vi "Read out VSET.vi"(4 "get more?":bool, 5 "All Channels (T)":bool=TRUE, 7 "Channel":u8, 8 "error in (no error)":errorcluster, 11 "BoardHandle":T2) -> (0 "error out":errorcluster, 1 "VSet constants":T1(array[cluster]), 2 "Vset values (V)":dbl[](array[numeric]) format="%.1f", 3 "BoardHandle out":T2)   [LabVIEW 2020, in "CAEN PSM.lvlib"]
doc: "This function returns VSet value"
uses:
  CAEN PSM.lvlib
  Private/BoardHandle.ctl
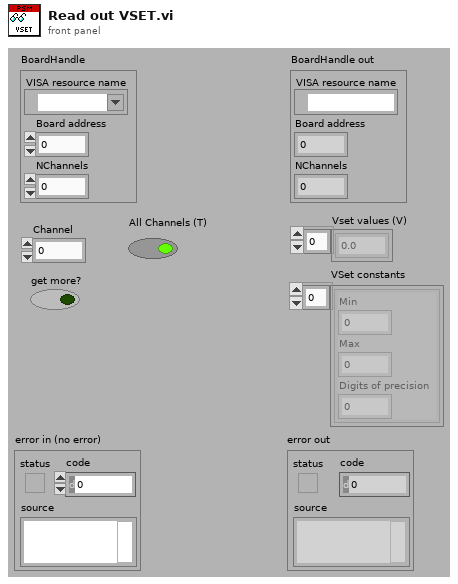
[diagram p1: front panel]
types:
  T1 = cluster{"Min":dbl, "Max":dbl, "Digits of precision":i32}[]
  T2 = typedef "CAEN PSM.lvlib/BoardHandle.ctl" = cluster{"VISA resource name":refnum<visa-resource-name>, "Board address":i8, "NChannels":u8}
  T3 = cluster{"Min":dbl, "Max":dbl, "Digits of precision":i32}
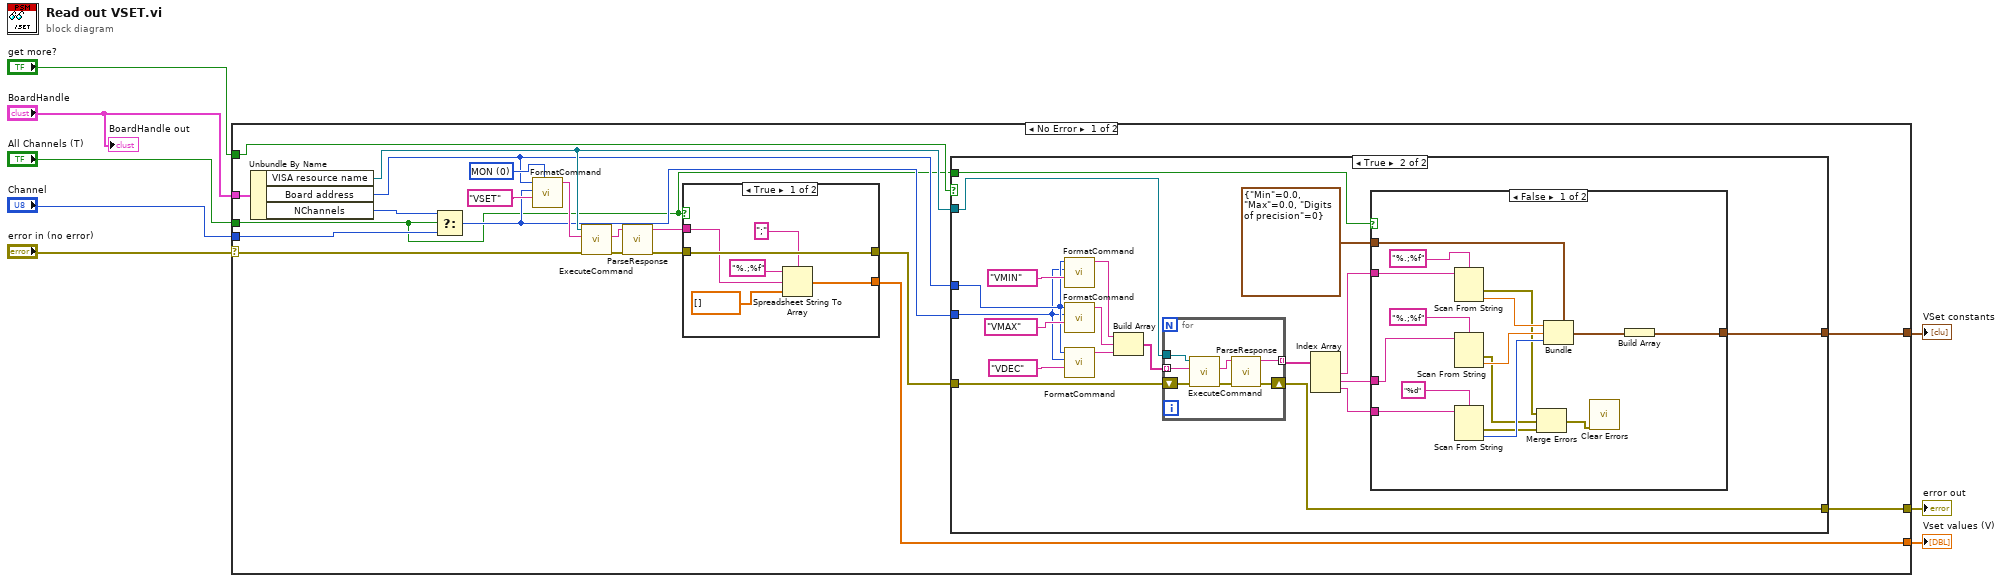
[diagram p0: block diagram]
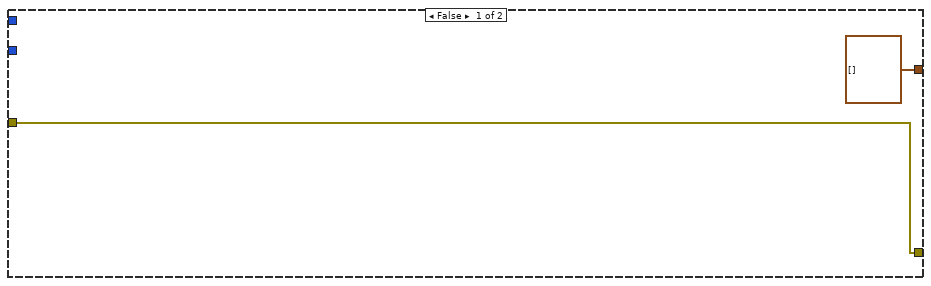
[diagram p2: hidden frame]
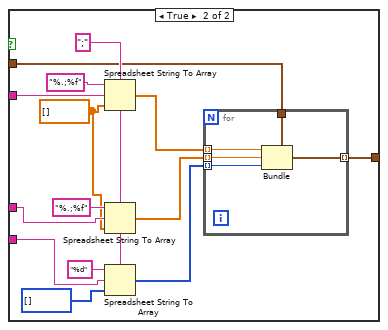
[diagram p3: hidden frame]
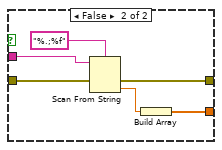
[diagram p4: hidden frame]
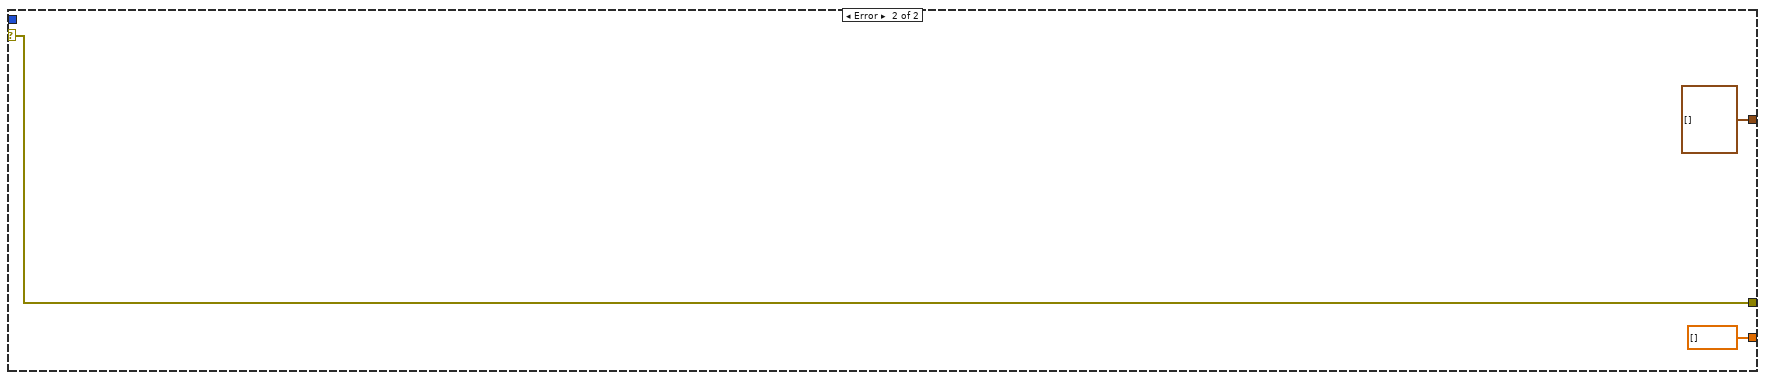
[diagram p5: hidden frame]
diagram:
  n1 = case shown="No Error" "error in (no error)" {
    selector: "error in (no error)" -> [w22 w106]
    tunnel: "All Channels (T)" -> [w9 _]
    tunnel: "Channel" -> [w27 _]
    tunnel: [w14 w106] -> w5
    tunnel: "BoardHandle" -> [w23 _]
    tunnel: [w17 dbl[] [] ("Trip value(s) s")] -> w3
    tunnel: "get more?" -> [w16 _]
    tunnel: [w10 T1 []] -> w1
    frame No Error {
      w28 = u8 0 items=["MON", "SET"] ("CMD")
      n2 = Unbundle By Name(w23) -> ("VISA resource name"=w13:refnum<visa-resource-name>, "Board address"=w12:i8, "NChannels"=w20:u8)
      n3 = Select(t=w20, s=w9, f=w27) -> (s? t:f=w11:u8)
      n4 = call "FormatCommand.vi"("CMD (MON)"=w28, "PAR"="VSET", "CH"=w11, "BD (0)"=w12) -> ("cmd"=w26:string)  [unwired: 7 in]
      n5 = call "ExecuteCommand.vi"("error in (no error)"=w22, "Command"=w26, "VISA resource name"=w13) -> ("error out"=w25:errorcluster, "Response"=w24:string)  [unwired: 6 in, 1 out]
      n6 = call "ParseResponse.vi"("error in (no error)"=w25, "Response"=w24) -> ("error out"=w18:errorcluster, "val"=w19:string)  [unwired: 6 in, 2 out]
      n7 = case shown="True" w9 {
        tunnel: w19 -> [w93 w103]
        tunnel: w18 -> [w97 w101]
        tunnel: [w97 w100] -> w15
        tunnel: [w96 w98] -> w17
        frame True {
          n8 = Spreadsheet String To Array(delimiter (Tab)=";", format string="%.;%f", spreadsheet string=w93, array type (2D Dbl)=dbl[] []) -> (array=w96:dbl[])
        }
        frame False {
          n9 = Scan From String(format string="%.;%f", input string=w103, error in=w101) -> (error out=w100:errorcluster, output 1=w99:dbl)  [unwired: 2 in, 2 out]
          n10 = Build Array(w99) -> (w98:dbl[])
        }
      }
      n11 = case shown="True" w16 {
        tunnel: w15 -> [w30 w41]
        tunnel: [w30 w40] -> w14
        tunnel: w13 -> [_ w44]
        tunnel: w12 -> [_ w43]
        tunnel: w11 -> [_ w42]
        tunnel: [T1 [] w34] -> w10
        tunnel: w9 -> [_ w31]
        frame False {
        }
        frame True {
          n12 = call "FormatCommand.vi"("PAR"="VMIN", "CH"=w42, "BD (0)"=w43) -> ("cmd"=w33:string)  [unwired: 8 in]
          n13 = call "FormatCommand.vi"("PAR"="VMAX", "CH"=w42, "BD (0)"=w43) -> ("cmd"=w32:string)  [unwired: 8 in]
          n14 = call "FormatCommand.vi"("PAR"="VDEC", "CH"=w42, "BD (0)"=w43) -> ("cmd"=w45:string)  [unwired: 8 in]
          n15 = Build Array(w33, w32, w45) -> (w46:string[])
          n16 = for {
            tunnel: w46 -> [w91] mode=indexing
            tunnel: w44 -> [w90]
            shift-right: [w88] -> w40
            shift-left: w41 -> [w89]
            tunnel: [w85] -> w39 mode=indexing
            n17 = call "ExecuteCommand.vi"("error in (no error)"=w89, "Command"=w91, "VISA resource name"=w90) -> ("error out"=w87:errorcluster, "Response"=w86:string)  [unwired: 6 in, 1 out]
            n18 = call "ParseResponse.vi"("error in (no error)"=w87, "Response"=w86) -> ("error out"=w88:errorcluster, "val"=w85:string)  [unwired: 6 in, 2 out]
          }
          n19 = Index Array(array=w39) -> (element #1=w38:string, element #2=w37:string, element #3=w36:string)  [unwired: 3 in]
          n20 = case shown="False" w31 {
            tunnel: w38 -> [w65 w78]
            tunnel: w37 -> [w60 w73]
            tunnel: w36 -> [w61 w74]
            tunnel: T3 {"Min"=0.0, "Max"=0.0, "Digits of precision"=0} -> [w59 w70]
            tunnel: [w54 w66] -> w34
            frame False {
              n21 = Scan From String(format string="%.;%f", input string=w65) -> (error out=w53:errorcluster, output 1=w58:dbl)  [unwired: 3 in, 2 out]
              n22 = Scan From String(format string="%.;%f", input string=w60) -> (error out=w52:errorcluster, output 1=w57:dbl)  [unwired: 3 in, 2 out]
              n23 = Scan From String(format string="%d", input string=w61) -> (error out=w51:errorcluster, output 1=w56:i32)  [unwired: 3 in, 2 out]
              n24 = Merge Errors(w53, w52, w51) -> (w50:errorcluster)
              n25 = Bundle(cluster=w59, "Min"=w58, "Max"=w57, "Digits of precision"=w56) -> (w55:T3)
              n26 = call <vilib>:"Clear Errors.vi"("error in (no error)"=w50) -> ()  [unwired: 5 in, 2 out]
              n27 = Build Array(w55) -> (w54:T1)
            }
            frame True {
              w72 = dbl[] [] ("array type (2D Dbl)")
              w75 = ";" ("delimiter (Tab)")
              n28 = Spreadsheet String To Array(delimiter (Tab)=w75, format string="%.;%f", spreadsheet string=w78, array type (2D Dbl)=w72) -> (array=w69:dbl[])
              n29 = Spreadsheet String To Array(delimiter (Tab)=w75, format string="%.;%f", spreadsheet string=w73, array type (2D Dbl)=w72) -> (array=w68:dbl[])
              n30 = Spreadsheet String To Array(delimiter (Tab)=w75, format string="%d", spreadsheet string=w74, array type (2D Dbl)=i32[] []) -> (array=w67:i32[])
              n31 = for {
                tunnel: w70 -> [w84]
                tunnel: w69 -> [w83] mode=indexing
                tunnel: w68 -> [w81] mode=indexing
                tunnel: w67 -> [w82] mode=indexing
                tunnel: [w80] -> w66 mode=indexing
                n32 = Bundle(cluster=w84, "Min"=w83, "Max"=w81, "Digits of precision"=w82) -> (w80:T3)
              }
            }
          }
        }
      }
    }
    frame Error {
    }
  }
  "error out" <- w5
  "Vset values (V)" <- w3
  "VSet constants" <- w1
  "BoardHandle out" <- "BoardHandle"
